vi "XNET System Close.vi"(11 "error in (no error)":errorcluster) -> (15 "error out":errorcluster)   [LabVIEW 2018]
doc: "Closes the XNET system to refresh XNET hardware information."
uses:
  nixlvapi.dll
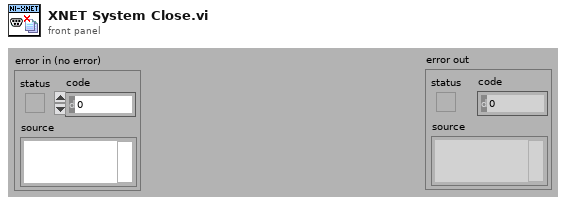
[diagram p1: front panel]
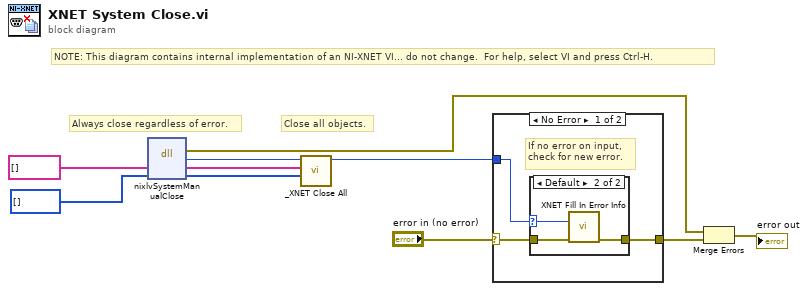
[diagram p0: block diagram]
diagram:
  # "Close all objects."
  # "Always close regardless of error."
  # "NOTE: This diagram contains internal implementation of an NI-XNET VI... do not change.  For help, select VI and press Ctrl-H."
  n1 = dll-call lib="nixlvapi.*" fn="nixlvSystemManualClose"("allNames"=string[] [] ("array of alias"), "allClasses"=u32[] [] ("array of alias")) -> (error out=w1:errorcluster, "return type"=w6:i32, "allNames"=w5:string[], "allClasses"=w4:u32[])  [unwired: 3 in, 1 out]
  n2 = call "_XNET Close All.vi"("all classes"=w4, "all names"=w5, "status code in"=w6) -> ("status code out"=w3:i32)  [unwired: 7 out]
  n3 = case shown="No Error" "error in (no error)" {
    selector: "error in (no error)" -> [w12 w18]
    tunnel: [w13 w18] -> w10
    tunnel: w3 -> [w11 _]
    frame No Error {
      # "If no error on input, \ncheck for new error."
      n4 = case shown="Default" w11 {
        selector: w11 -> [_ w15]
        tunnel: w12 -> [w14 w16]
        tunnel: [w14 w17] -> w13
        frame 0 {
        }
        frame Default {
          n5 = call "XNET Fill In Error Info.vi"("status code"=w15, "error in"=w16) -> ("error out"=w17:errorcluster)  [unwired: 13 out]
        }
      }
    }
    frame Error {
    }
  }
  n6 = Merge Errors(w1, w10) -> (→"error out":errorcluster)
